vi "Load Config.vi"(8 "error in (no error)":errorcluster, 11 "IEPEChannel in":refnum<class "IEPEChannel.lvclass">) -> (0 "error out":errorcluster, 3 "IEPEChannel out":refnum<class "IEPEChannel.lvclass">)   [LabVIEW 2020, in "VolatusDAQConfig.lvlib" / "IEPEChannel.lvclass"]
uses:
  IEPEChannel.lvclass
  IEPEChannel.lvclass/IEPEChannel.ctl
  VolatusConfig/VolatusConfigElement/VolatusConfigElement.lvclass
  lv-cdm/CDM-Config/Config Element/Config Element.lvclass
  C:/dev/lv20CE/relink/lv-volatus/VolatusDAQConfig/DAQmxChannel/DAQmxChannel.lvclass
  C:/dev/lv20CE/relink/lv-volatus/VolatusConfig/Channel/Channel.lvclass
  C:/dev/lv20CE/relink/lv-volatus/VolatusConfig/VolatusConfigElement/VolatusConfigElement.lvclass
  C:/dev/lv20CE/relink/lv-volatus/VolatusDAQConfig/IEPEChannel/IEPEChannel.lvclass
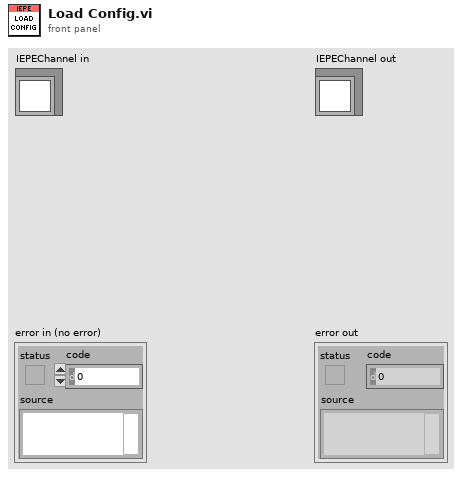
[diagram p1: front panel]
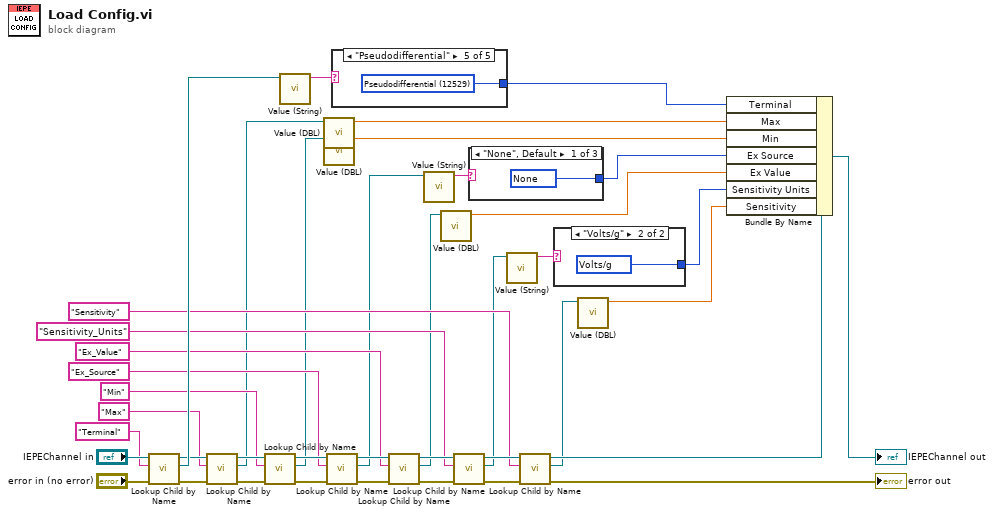
[diagram p0: block diagram]
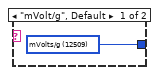
[diagram p2: hidden frame]
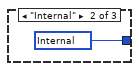
[diagram p3: hidden frame]
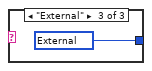
[diagram p4: hidden frame]
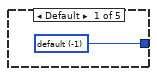
[diagram p5: hidden frame]
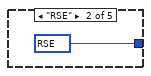
[diagram p6: hidden frame]
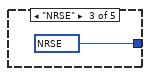
[diagram p7: hidden frame]
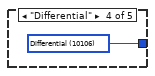
[diagram p8: hidden frame]
diagram:
  n1 = call "Lookup Child by Name.vi"("error in (no error)"="error in (no error)", "Child Name"="Terminal", "VolatusConfigElement in"="IEPEChannel in") -> ("error out"=w32:errorcluster, "Child"=w35:refnum<class "Config Element.lvclass">, "VolatusConfigElement out"=w34:refnum<class "IEPEChannel.lvclass">)  [unwired: 5 in, 1 out]
  n2 = call "Lookup Child by Name.vi"("error in (no error)"=w32, "Child Name"="Max", "VolatusConfigElement in"=w34) -> ("error out"=w30:errorcluster, "Child"=w13:refnum<class "Config Element.lvclass">, "VolatusConfigElement out"=w31:refnum<class "IEPEChannel.lvclass">)  [unwired: 5 in, 1 out]
  n3 = call "Lookup Child by Name.vi"("error in (no error)"=w30, "Child Name"="Min", "VolatusConfigElement in"=w31) -> ("error out"=w27:errorcluster, "Child"=w12:refnum<class "Config Element.lvclass">, "VolatusConfigElement out"=w28:refnum<class "IEPEChannel.lvclass">)  [unwired: 5 in, 1 out]
  n4 = call "Value (String).vi"("Config Element in"=w35) -> ("String Value"=w37:string)  [unwired: 9 in, 1 out]
  n5 = call "Value (DBL).vi"("Config Element in"=w13) -> ("DBL Value"=w14:dbl)  [unwired: 9 in, 1 out]
  n6 = call "Value (DBL).vi"("Config Element in"=w12) -> ("DBL Value"=w11:dbl)  [unwired: 9 in, 1 out]
  n7 = call "Lookup Child by Name.vi"("error in (no error)"=w27, "Child Name"="Ex_Source", "VolatusConfigElement in"=w28) -> ("error out"=w24:errorcluster, "Child"=w9:refnum<class "Config Element.lvclass">, "VolatusConfigElement out"=w25:refnum<class "IEPEChannel.lvclass">)  [unwired: 5 in, 1 out]
  n8 = case shown="\"Pseudodifferential\"" w37 {
    tunnel: [w42 w43 w44 w45 w46] -> w36
    frame Default {
      w42 = -1 items=["default"=-1, "RSE"=10083, "NRSE"=10078, "Differential"=10106, "Pseudodifferential"=12529] ("Terminal")
    }
    frame "RSE" {
      w43 = 10083 items=["default"=-1, "RSE"=10083, "NRSE"=10078, "Differential"=10106, "Pseudodifferential"=12529] ("Terminal")
    }
    frame "NRSE" {
      w44 = 10078 items=["default"=-1, "RSE"=10083, "NRSE"=10078, "Differential"=10106, "Pseudodifferential"=12529] ("Terminal")
    }
    frame "Differential" {
      w45 = 10106 items=["default"=-1, "RSE"=10083, "NRSE"=10078, "Differential"=10106, "Pseudodifferential"=12529] ("Terminal")
    }
    frame "Pseudodifferential" {
      w46 = 12529 items=["default"=-1, "RSE"=10083, "NRSE"=10078, "Differential"=10106, "Pseudodifferential"=12529] ("Terminal")
    }
  }
  n9 = call "Lookup Child by Name.vi"("error in (no error)"=w24, "Child Name"="Ex_Value", "VolatusConfigElement in"=w25) -> ("error out"=w21:errorcluster, "Child"=w7:refnum<class "Config Element.lvclass">, "VolatusConfigElement out"=w22:refnum<class "IEPEChannel.lvclass">)  [unwired: 5 in, 1 out]
  n10 = call "Value (String).vi"("Config Element in"=w9) -> ("String Value"=w10:string)  [unwired: 9 in, 1 out]
  n11 = call "Value (DBL).vi"("Config Element in"=w7) -> ("DBL Value"=w6:dbl)  [unwired: 9 in, 1 out]
  n12 = call "Lookup Child by Name.vi"("error in (no error)"=w21, "Child Name"="Sensitivity_Units", "VolatusConfigElement in"=w22) -> ("error out"=w18:errorcluster, "Child"=w3:refnum<class "Config Element.lvclass">, "VolatusConfigElement out"=w19:refnum<class "IEPEChannel.lvclass">)  [unwired: 5 in, 1 out]
  n13 = case shown="\"None\", Default" w10 {
    tunnel: [w47 w48 w49] -> w8
    frame "None", Default {
      w47 = 10230 items=["Internal"=10200, "External"=10167, "None"=10230] ("Ex Source")
    }
    frame "Internal" {
      w48 = 10200 items=["Internal"=10200, "External"=10167, "None"=10230] ("Ex Source")
    }
    frame "External" {
      w49 = 10167 items=["Internal"=10200, "External"=10167, "None"=10230] ("Ex Source")
    }
  }
  n14 = call "Value (String).vi"("Config Element in"=w3) -> ("String Value"=w2:string)  [unwired: 9 in, 1 out]
  n15 = call "Lookup Child by Name.vi"("error in (no error)"=w18, "Child Name"="Sensitivity", "VolatusConfigElement in"=w19) -> ("error out"=→"error out":errorcluster, "Child"=w5:refnum<class "Config Element.lvclass">, "VolatusConfigElement out"=w16:refnum<class "IEPEChannel.lvclass">)  [unwired: 5 in, 1 out]
  n16 = case shown="\"Volts/g\"" w2 {
    tunnel: [w50 w51] -> w1
    frame "mVolt/g", Default {
      w50 = 12509 items=["mVolts/g"=12509, "Volts/g"=12510] ("Sensitivity Units")
    }
    frame "Volts/g" {
      w51 = 12510 items=["mVolts/g"=12509, "Volts/g"=12510] ("Sensitivity Units")
    }
  }
  n17 = call "Value (DBL).vi"("Config Element in"=w5) -> ("DBL Value"=w4:dbl)  [unwired: 9 in, 1 out]
  n18 = Bundle By Name(cluster=w16, "Terminal"=w36, "Max"=w14, "Min"=w11, "Ex Source"=w8, "Ex Value"=w6, "Sensitivity Units"=w1, "Sensitivity"=w4) -> (→"IEPEChannel out":refnum<class "IEPEChannel.lvclass">)
